vi "SetValue.vi"(8 "error in":errorcluster, 10 "Value":string, 11 "CustomElement in":refnum<class "CustomElement.lvclass">) -> (0 "error out":errorcluster, 3 "CustomElement out":refnum<class "CustomElement.lvclass">)   [LabVIEW 2021, in "ProligentXMLGenerator.lvlib" / "CustomElement.lvclass"]
doc: "This value need to be formated as a valid XML element."
uses:
  CustomElement.lvclass
  CustomElement.lvclass/CustomElement.ctl
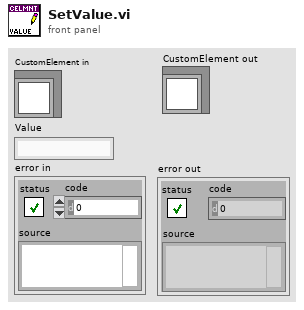
[diagram p1: front panel]
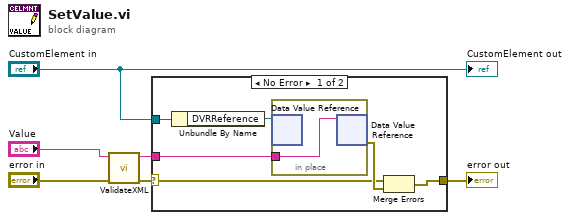
[diagram p0: block diagram]
diagram:
  n1 = call "ValidateXML.vi"("error in"="error in", "Value in"="Value") -> ("error out"=w2:errorcluster, "Value out"=w1:string)  [unwired: 8 in]
  n2 = case shown="No Error" w2 {
    selector: w2 -> [w8 w14]
    tunnel: [w11 w14] -> w4
    tunnel: "CustomElement in" -> [w10 _]
    tunnel: w1 -> [w7 _]
    frame No Error {
      n3 = Unbundle By Name(w10) -> ("DVRReference"=w9:refnum<data-value>)
      n4 = in-place "In Place Element Structure" {
        in-place-border: w7 -> [w13]
        n5 = in-place-dvr #1(w9) -> ()  [unwired: 2 out]
        n6 = in-place-dvr #1(w13) -> (w12:errorcluster)  [unwired: 1 out]
      }
      n7 = Merge Errors(w8, w12) -> (w11:errorcluster)
    }
    frame Error {
    }
  }
  "error out" <- w4
  "CustomElement out" <- "CustomElement in"
